vi "TSPopup.Breakout Controls to Register.vi"(11 "Popup":refnum<vi>) -> (1 "Color & Ring":refnum<vi>[](array[refnum]), 3 "Unknown":refnum<vi>, 4 "Clusters OK":refnum<vi>[](array[refnum]), 6 "Clusters Cancel":refnum<vi>[](array[refnum]))   [LabVIEW 2016, in "TSPopup.lvlib" / "TSPopup.lvclass"]
doc: "Get references of popout cluster pieces to monitor events for.\n\nType Sensitive Popup \nCopyright © 2007, J. David Saunders\nAll rights reserved."
uses:
  <userlib>/TSPopup/TSPopup.lvclass
  <userlib>/TSPopup/TSPopup.Data Type.ctl
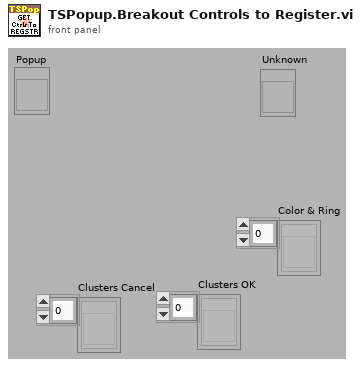
[diagram p1: front panel]
types:
  T1 = typedef "TSPopup.lvlib/TSPopup.lvclass/TSPopup.Data Type.ctl" = enum16{"Unkown", "NO POPUP", "String", "Integer", "Float", "Color", "Boolean", "Ring", "Captioned String", "Captioned Integer", "Button Color", "2 Int Cluster", "4 Int Cluster", "check"}
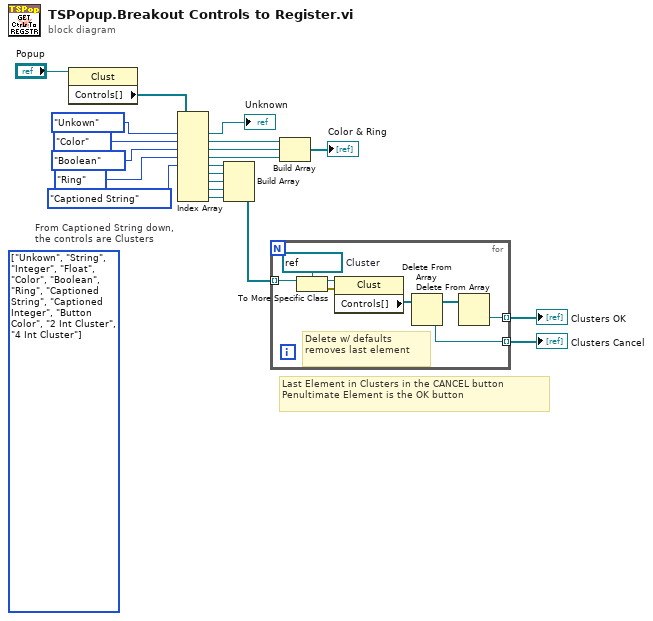
[diagram p0: block diagram]
diagram:
  (unwired) T1[] [enum."Unkown", enum."String", enum."Integer", enum."Float", enum."Color", enum."Boolean", enum."Ring", enum."Captioned String", enum."Captioned Integer", enum."Button Color", enum."2 Int Cluster", enum."4 Int Cluster"] items=["Unkown", "NO POPUP", "String", "Integer", "Float", "Color", "Boolean", "Ring", "Captioned String", "Captioned Integer", "Button Color", "2 Int Cluster", "4 Int Cluster", "check"]
  # "Last Element in Clusters in the CANCEL button\nPenultimate Element is the OK button"
  # "From Captioned String down,\nthe controls are Clusters"
  n1 = property class="Clust"(reference="Popup") -> ("Controls[]"=w19:refnum<vi>[])  [unwired: 1 in, 2 out]
  n2 = Index Array(array=w19, index #1=TSPopup.Data_Type."Unkown" ("Prop Type"), index #2=TSPopup.Data_Type."Color" ("Prop Type"), index #3=TSPopup.Data_Type."Boolean" ("Prop Type"), index #4=TSPopup.Data_Type."Ring" ("Prop Type"), index #5=TSPopup.Data_Type."Captioned String" ("Prop Type")) -> (element #1=→"Unknown":refnum<vi>, element #2=w2:refnum<vi>, element #3=w17:refnum<vi>, element #4=w16:refnum<vi>, element #5=w14:refnum<vi>, element #6=w13:refnum<vi>, element #7=w12:refnum<vi>, element #8=w11:refnum<vi>, element #9=w10:refnum<vi>)  [unwired: 4 in]
  n3 = Build Array(w14, w13, w12, w11, w10) -> (w9:refnum<vi>[])
  n4 = for {
    tunnel: w9 -> [w28] mode=indexing
    tunnel: [w23] -> w7 mode=indexing
    tunnel: [w21] -> w8 mode=indexing
    w27 = refnum<vi> refnum  # Cluster
    # "Delete w/ defaults\nremoves last element"
    n5 = To More Specific Class(target class=w27, reference=w28) -> (specific class reference=w26:refnum<vi>, error out=w25:errorcluster)  [unwired: 1 in]
    n6 = property class="Clust"(reference=w26, error in=w25) -> ("Controls[]"=w24:refnum<vi>[])  [unwired: 2 out]
    n7 = Delete From Array(array=w24) -> (deleted portion=w23:refnum<vi>, array with subset deleted=w22:refnum<vi>[])  [unwired: 2 in]
    n8 = Delete From Array(array=w22) -> (deleted portion=w21:refnum<vi>)  [unwired: 2 in, 1 out]
  }
  "Clusters OK" <- w8
  "Clusters Cancel" <- w7
  n9 = Build Array(w2, w17, w16) -> (→"Color & Ring":refnum<vi>[])
